vi "SigManipulationLJArrayTest.vi"(11 "Data":dbl[][](array[numeric])) -> (3 "Array":dbl[][](array[numeric]))   [LabVIEW 2021]
panel:
  out "error out":errorcluster
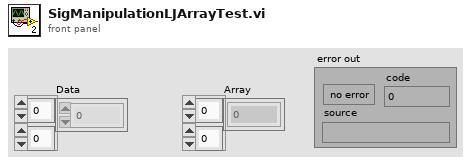
[diagram p1: front panel]
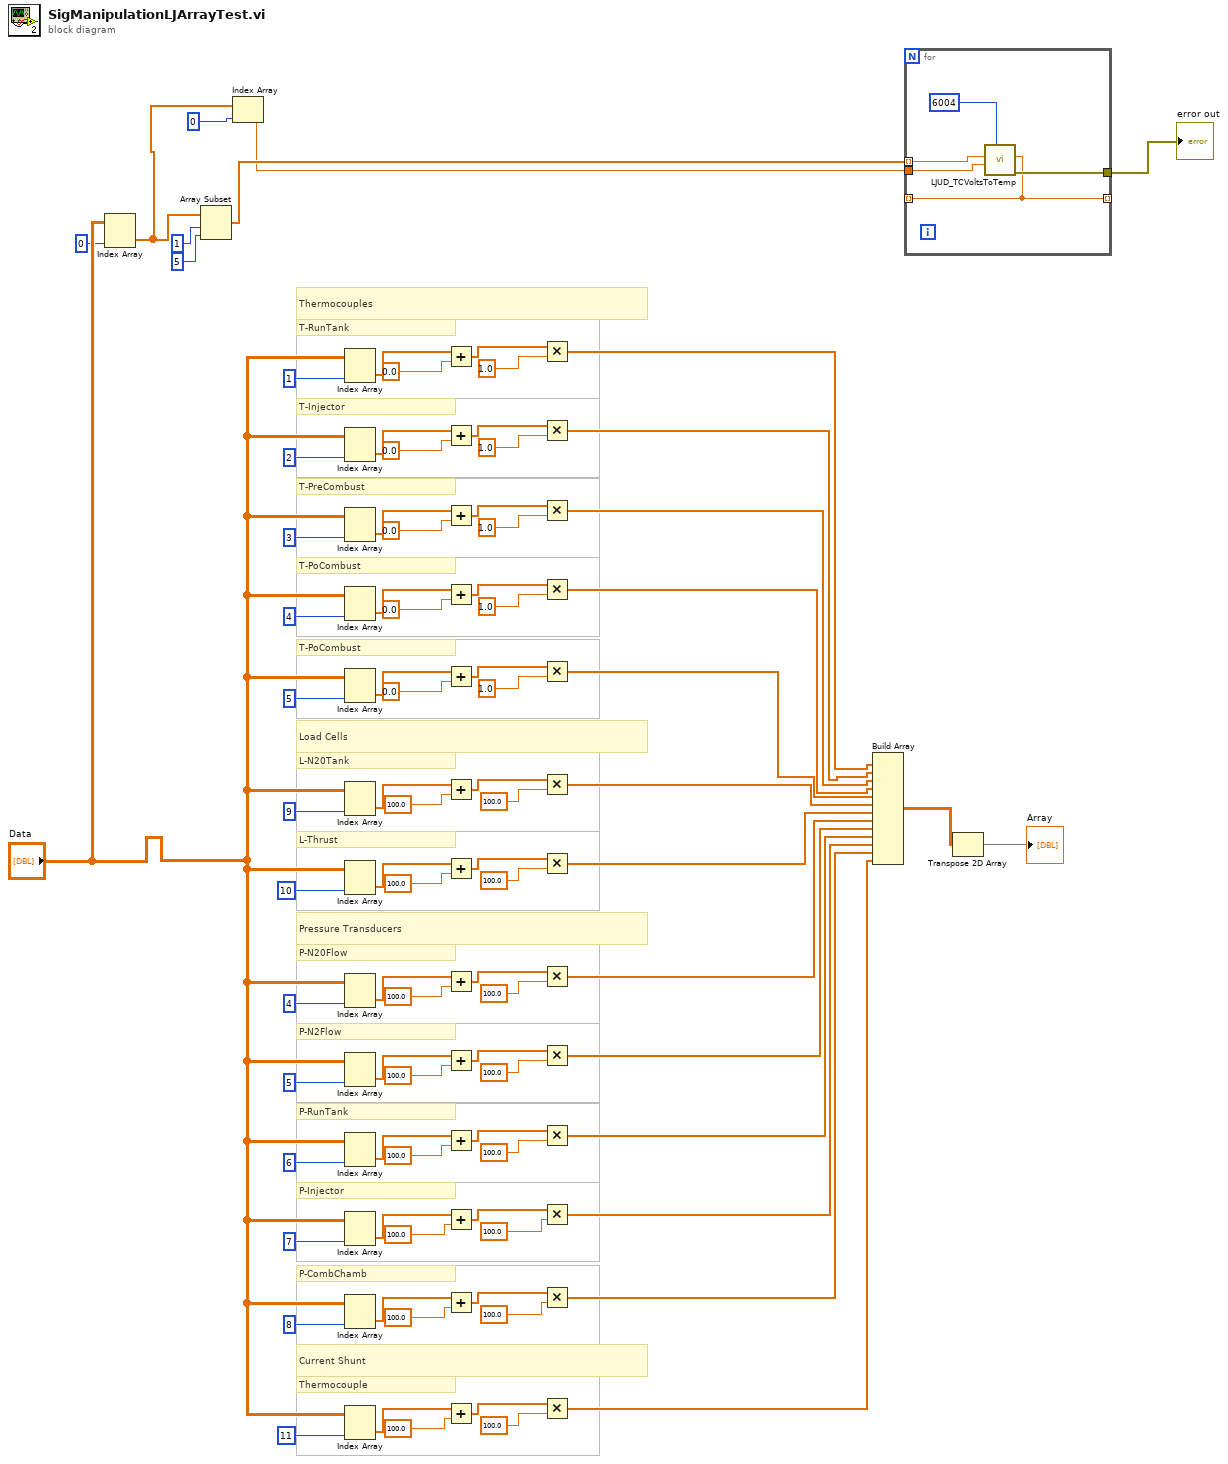
[diagram p0: block diagram]
diagram:
  # "T-PoCombust"
  # "P-CombChamb"
  # "Current Shunt"
  # "Thermocouple"
  # "P-Injector"
  # "P-RunTank"
  # "P-N2Flow"
  # "Pressure Transducers"
  # "P-N20Flow"
  # "L-Thrust"
  # "Load Cells"
  # "L-N20Tank"
  # "T-PoCombust"
  # "T-PreCombust"
  # "T-Injector"
  # "Thermocouples"
  # "T-RunTank"
  n1 = Index Array(array="Data", index (col)=0 ("disabled index (col)")) -> (element=w5:dbl[])  [unwired: 1 in]
  n2 = Array Subset(array=w5, index=1, length=5) -> (w9:dbl[])
  n3 = Index Array(array=w5, index=0 ("disabled index (col)")) -> (element=w8:dbl)
  n4 = Index Array(array="Data", index (col)=1) -> (element=w38:dbl[])  [unwired: 1 in]
  n5 = Index Array(array="Data", index (col)=2) -> (element=w37:dbl[])  [unwired: 1 in]
  n6 = Index Array(array="Data", index (col)=3) -> (element=w36:dbl[])  [unwired: 1 in]
  n7 = Index Array(array="Data", index (col)=4) -> (element=w35:dbl[])  [unwired: 1 in]
  n8 = Index Array(array="Data", index (col)=5) -> (element=w15:dbl[])  [unwired: 1 in]
  n9 = Index Array(array="Data", index (col)=9) -> (element=w34:dbl[])  [unwired: 1 in]
  n10 = Index Array(array="Data", index (col)=10) -> (element=w33:dbl[])  [unwired: 1 in]
  n11 = Index Array(array="Data", index (col)=4) -> (element=w32:dbl[])  [unwired: 1 in]
  n12 = Index Array(array="Data", index (col)=5) -> (element=w31:dbl[])  [unwired: 1 in]
  n13 = Index Array(array="Data", index (col)=6) -> (element=w30:dbl[])  [unwired: 1 in]
  n14 = Index Array(array="Data", index (col)=7) -> (element=w29:dbl[])  [unwired: 1 in]
  n15 = Index Array(array="Data", index (col)=8) -> (element=w26:dbl[])  [unwired: 1 in]
  n16 = Index Array(array="Data", index (col)=11) -> (element=w23:dbl[])  [unwired: 1 in]
  n17 = Add(x=w38, y=0.0) -> (x+y=w89:dbl[])
  n18 = Add(x=w37, y=0.0) -> (x+y=w86:dbl[])
  n19 = Add(x=w36, y=0.0) -> (x+y=w83:dbl[])
  n20 = Add(x=w35, y=0.0) -> (x+y=w80:dbl[])
  n21 = Add(x=w15, y=0.0) -> (x+y=w19:dbl[])
  n22 = Add(x=w34, y=100.0) -> (x+y=w77:dbl[])
  n23 = Add(x=w33, y=100.0) -> (x+y=w74:dbl[])
  n24 = Add(x=w32, y=100.0) -> (x+y=w71:dbl[])
  n25 = Add(x=w31, y=100.0) -> (x+y=w68:dbl[])
  n26 = Add(x=w30, y=100.0) -> (x+y=w65:dbl[])
  n27 = Add(x=w29, y=100.0) -> (x+y=w62:dbl[])
  n28 = Add(x=w26, y=100.0) -> (x+y=w49:dbl[])
  n29 = Add(x=w23, y=100.0) -> (x+y=w61:dbl[])
  n30 = Multiply(x=w89, y=1.0) -> (x*y=w14:dbl[])
  n31 = Multiply(x=w86, y=1.0) -> (x*y=w13:dbl[])
  n32 = Multiply(x=w83, y=1.0) -> (x*y=w12:dbl[])
  n33 = Multiply(x=w80, y=1.0) -> (x*y=w11:dbl[])
  n34 = Multiply(x=w19, y=1.0) -> (x*y=w10:dbl[])
  n35 = Multiply(x=w77, y=100.0) -> (x*y=w46:dbl[])
  n36 = Multiply(x=w74, y=100.0) -> (x*y=w45:dbl[])
  n37 = Multiply(x=w71, y=100.0) -> (x*y=w44:dbl[])
  n38 = Multiply(x=w68, y=100.0) -> (x*y=w43:dbl[])
  n39 = Multiply(x=w65, y=100.0) -> (x*y=w42:dbl[])
  n40 = Multiply(x=w62, y=100.0) -> (x*y=w41:dbl[])
  n41 = Multiply(x=w49, y=100.0) -> (x*y=w40:dbl[])
  n42 = Multiply(x=w61, y=100.0) -> (x*y=w39:dbl[])
  n43 = Build Array(w14, w13, w12, w11, w10, w46, w45, w44, w43, w42, w41, w40, w39) -> (w21:dbl[][])  [unwired: 1 in]
  n44 = for {
    tunnel: w9 -> [w94] mode=indexing
    tunnel: w8 -> [w93]
    tunnel: [w90] -> _ mode=indexing
    tunnel: [w91] -> w1
    tunnel: [w90] -> _ mode=indexing
    n45 = call "LJUD_TCVoltsToTemp.vi"("TCType"=6004, "CJTempK"=w93, "TCVolts"=w94) -> ("error out"=w91:errorcluster, "TCTempC"=w90:dbl)  [unwired: 5 in, 2 out]
  }
  "error out" <- w1
  n46 = Transpose 2D Array(2D array=w21) -> (transposed array=→"Array":dbl[][])
